vi "Server Generate ACK Event.vi"(8 "error in":errorcluster, 9 "ACK (True)":bool=TRUE, 10 "header":string, 11 "server event ref":refnum<vi>) -> (0 "error out":errorcluster)   [LabVIEW 2018]
doc: "Sends simple ACK no ACK answer event to server."
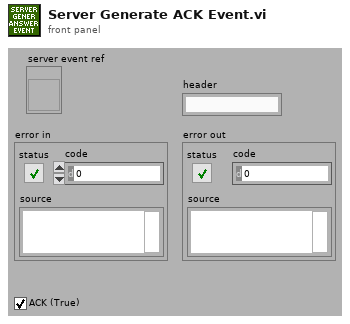
[diagram p1: front panel]
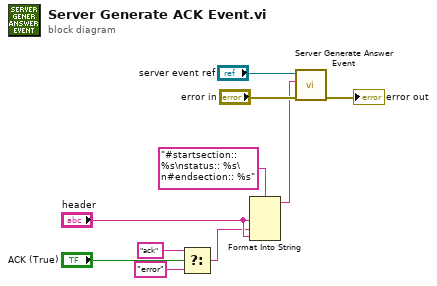
[diagram p0: block diagram]
diagram:
  n1 = Select(t="ack", s="ACK (True)", f="error") -> (s? t:f=w8:string)
  n2 = Format Into String(format string="#startsection:: %s\nstatus:: %s\n#endsection:: %s", "header", w8, "header") -> (resulting string=w1:string)  [unwired: 2 in, 1 out]
  n3 = call "Server Generate Answer Event.vi"("error in"="error in", "event data"=w1, "server event ref"="server event ref") -> ("error out"=→"error out":errorcluster)  [unwired: 8 in]
